vi "Create HTML.vi"(7 "FP Reference":refnum<class "Web Front Panel.lvclass">, 8 "error in (no error)":errorcluster, 10 "VI Identifier":string, 11 "Control In":refnum<class "Control.lvclass">) -> (0 "error out":errorcluster, 1 "js code for controls":string, 2 "js variables":string, 3 "Control Out":refnum<class "Control.lvclass">, 4 "script dependencies":string[](array[string]), 5 "HTML":string, 6 "js code for indicators":string)   [LabVIEW 2017, in "Front Panel Publisher.lvlib" / "Control.lvclass"]
uses:
  Control.lvclass
  Object_class/Object.lvclass
  Front Panel Publisher.lvlib
  Web Front Panel_class/Web Front Panel.lvclass
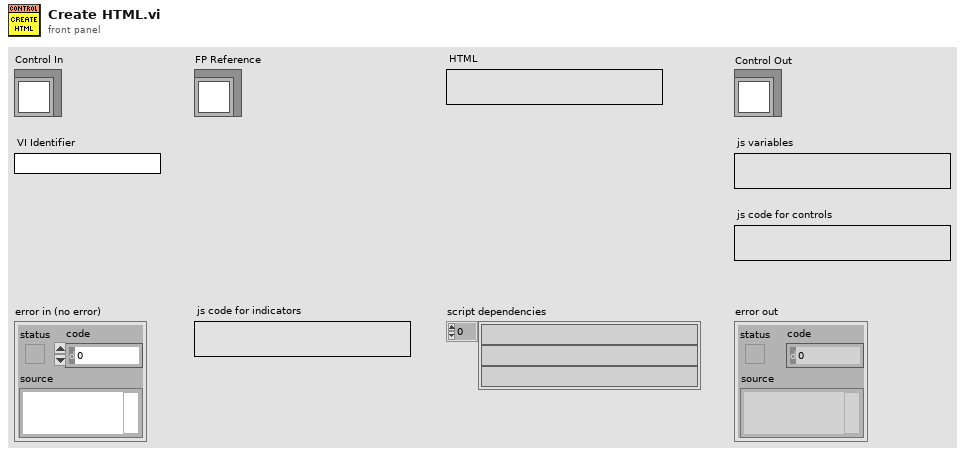
[diagram p1: front panel]
types:
  T1 = typedef "Front Panel Publisher.lvlib/Object.lvclass/Attributes.ctl" = cluster{"UID":i32, "Type":string, "Starting Location":T2, "Reference":refnum<vi>, "Cluster Component":bool, "Starting Rect Position":cluster{"Left":i16, "Top":i16}, "Owning Pane":refnum<vi>, "Master Total Rect Delta":T3}
  T2 = typedef "Front Panel Publisher.lvlib/Object.lvclass/Coordinates.ctl" = cluster{"Left":i32, "Top":i32, "Height":u32, "Width":u32}
  T3 = typedef "LVRectTypeDef.ctl" = cluster{"Left":i16, "Top":i16, "Right":i16, "Bottom":i16}
  T4 = typedef "Front Panel Publisher.lvlib/Control.lvclass/Attributes.ctl" = cluster{"Description":string, "Indicator":bool, "Default Value":variant, "Control Index":i32, "Label":refnum<class "Text.lvclass">, "Caption":refnum<class "Text.lvclass">, "Image b64":string, "No Control Index":bool, "Display Mode":T5}
  T5 = typedef "Front Panel Publisher.lvlib/Web Front Panel.lvclass/Enum - Control Display Mode.ctl" = enum16{"Value Only", "Value and Visibility", "Boolean Value Only", "Boolean Value and Visibility", "Control is Image", "Image and Visibility"}
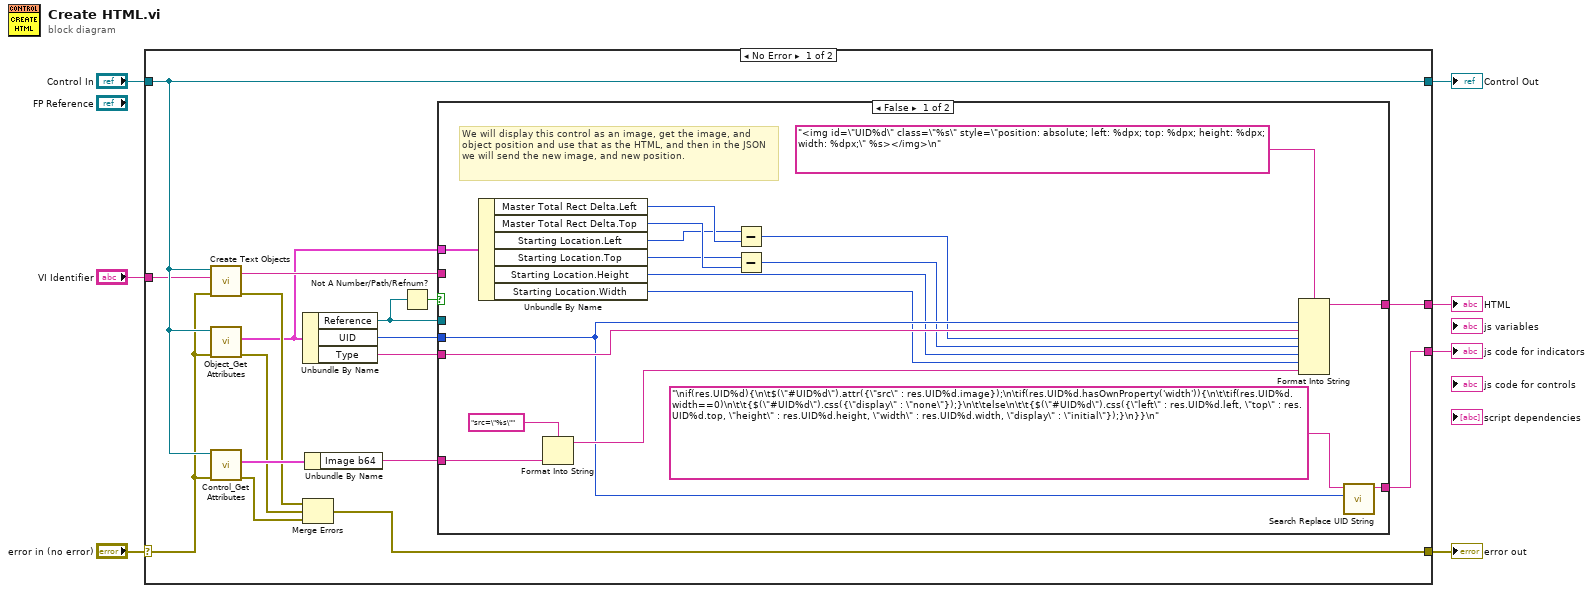
[diagram p0: block diagram]
diagram:
  n1 = case shown="No Error" "error in (no error)" {
    selector: "error in (no error)" -> [w20 w45]
    tunnel: [w14 w45] -> w6
    tunnel: [w21 w44] -> w4
    tunnel: "Control In" -> [w21 w44]
    tunnel: [w23 _] -> w3
    tunnel: [w15 _] -> w2
    tunnel: "VI Identifier" -> [w13 _]
    frame No Error {
      n2 = call-dynamic "Create Text Objects.vi"("error in (no error)"=w20, "VI Name"=w13, "Control In"=w21) -> ("error out"=w19:errorcluster, "HTML"=w11:string)  [unwired: 5 in, 2 out]
      n3 = call "Object_Get Attributes.vi"("error in (no error)"=w20, "Object In"=w21) -> ("error out"=w18:errorcluster, "Object Attributes"=w8:T1)  [unwired: 7 in, 1 out]
      n4 = call "Control_Get Attributes.vi"("error in (no error)"=w20, "Control In"=w21) -> ("error out"=w17:errorcluster, "Control Attributes"=w22:T4)  [unwired: 7 in, 1 out]
      n5 = Unbundle By Name(w8) -> ("Reference"=w10:refnum<vi>, "UID"=w12:i32, "Type"=w24:string)
      n6 = Merge Errors(w19, w18, w17) -> (w14:errorcluster)
      n7 = Unbundle By Name(w22) -> ("Image b64"=w16:string)
      n8 = Not A Number/Path/Refnum?(number/path/refnum=w10) -> (NaN/Path/Refnum?=w9:bool)
      n9 = case shown="False" w9 {
        tunnel: w24 -> [w42 _]
        tunnel: [w41 w43] -> w23
        tunnel: w16 -> [w40 _]
        tunnel: [w39 _] -> w15
        tunnel: w12 -> [w35 _]
        tunnel: w10 -> [_ _]
        tunnel: w11 -> [_ w43]
        tunnel: w8 -> [w33 _]
        frame False {
          # "We will display this control as an image, get the image, and object position and use that as the HTML, and then in the JSON we will send the new image, and new position."
          n10 = Unbundle By Name(w33) -> ("Master Total Rect Delta.Left"=w30:i16, "Master Total Rect Delta.Top"=w29:i16, "Starting Location.Left"=w27:i32, "Starting Location.Top"=w28:i32, "Starting Location.Height"=w32:u32, "Starting Location.Width"=w31:u32)
          n11 = Format Into String(format string="src=\"%s\"", w40) -> (resulting string=w37:string)  [unwired: 2 in, 1 out]
          n12 = Subtract(x=w27, y=w30) -> (x-y=w25:i32)
          n13 = Subtract(x=w28, y=w29) -> (x-y=w26:i32)
          n14 = Format Into String(format string="<img id=\"UID%d\" class=\"%s\" style=\"position: absolute; left: %dpx; top: %dpx; height: %dpx; width: %dpx;\" %s></img>\n", w35, w42, w25, w26, w32, w31, w37) -> (resulting string=w41:string)  [unwired: 2 in, 1 out]
          n15 = call "Search Replace UID String.vi"("UID"=w35, "Input String"="\nif(res.UID%d){\n\t$(\"#UID%d\").attr({\"src\" : res.UID%d.image});\n\tif(res.UID%d.hasOwnProperty('width')){\n\t\tif(res.UID%d.width==0)\n\t\t{$(\"#UID%d\").css({\"display\" : \"none\"});}\n\t\telse\n\t\t{$(\"#UID%d\").css({\"left\" : res.UID%d.left, \"top\" : res.UID%d.top, \"height\" : res.UID%d.height, \"width\" : res.UID%d.width, \"display\" : \"initial\"});}\n}}\n") -> ("Output String"=w39:string)  [unwired: 9 in]
        }
        frame True {
          # "If the control reference is invalid, we may have some free labels that still can be displayed."
        }
      }
    }
    frame Error {
    }
  }
  "error out" <- w6
  "Control Out" <- w4
  "HTML" <- w3
  "js code for indicators" <- w2
